vi "Size of Largest Finite Area.vi"(10 "Closest Point Indices in":i32[][](array[numeric]), 11 "Finite Regions":i32[](array[numeric])) -> (3 "Numeric":i16)   [LabVIEW 2019]
doc: "Find largest, finite region. By this point, all infinite spaces should be set to -1."
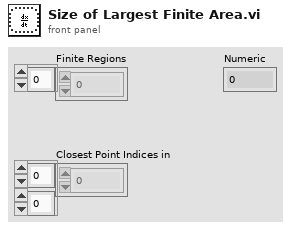
[diagram p1: front panel]
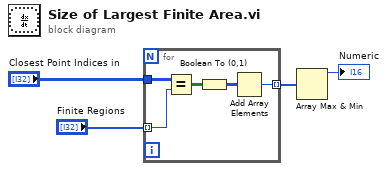
[diagram p0: block diagram]
diagram:
  n1 = for {
    tunnel: "Finite Regions" -> [w6] mode=indexing
    tunnel: "Closest Point Indices in" -> [w5]
    tunnel: [w7] -> w2 mode=indexing
    n2 = Equal?(x=w5, y=w6) -> (x = y?=w9:bool[][])
    n3 = Boolean To (0,1)(Boolean=w9) -> (0, 1=w8:i16[][])
    n4 = Add Array Elements(numeric array=w8) -> (sum=w7:i16)
  }
  n5 = Array Max & Min(array=w2) -> (max value=→"Numeric":i16)  [unwired: 3 out]
